vi "Put_Tracks_To_FRM-FRM_Matrix-3.vi"(2 "error IN":errorcluster, 3 "[IN] Matrix for Estimation \nSizes of Frame-to-Frame \nDisplacements from Tracks":dbl[][](array[numeric]), 5 "[IN] Tracks w/t Problems":T1(array[cluster])) -> (0 "error OUT":errorcluster, 1 "[OUT] Frame-to-Frame\nDisplacements Extract\nFrom Tracks":dbl[][](array[numeric]))   [LabVIEW 2013]
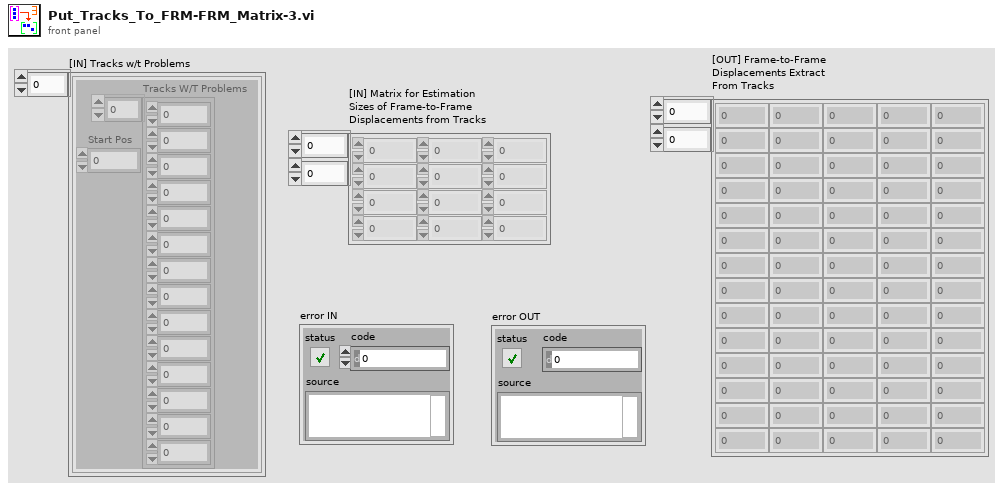
[diagram p1: front panel]
types:
  T1 = cluster{"Tracks W/T Problems":dbl[], "Start Pos":i32}[]
  T2 = cluster{"Tracks W/T Problems":dbl[], "Start Pos":i32}
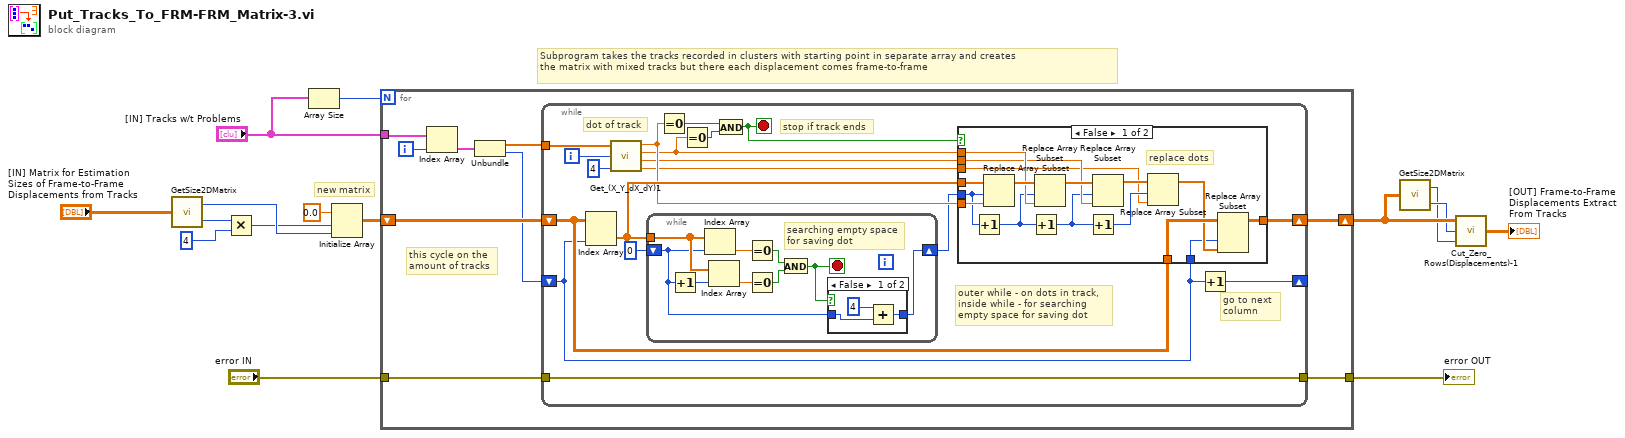
[diagram p0: block diagram]
diagram:
  # "Subprogram takes the tracks recorded in clusters with starting point in separate array and creates \nthe matrix with mixed tracks but there each displacement comes frame-to-frame"
  # "new matrix"
  n1 = call "GetSize2DMatrix.vi"("Array IN (2D)"="[IN] Matrix for Estimation \nSizes of Frame-to-Frame \nDisplacements from Tracks") -> ("# Cols"=w4:i32, "# Rows"=w3:i32)
  n2 = Multiply(x=w3, y=4 ("x")) -> (x*y=w1:i32)
  n3 = Array Size(array="[IN] Tracks w/t Problems") -> (size(s)=w8:i32)
  n4 = Initialize Array(0.0 ("element"), w1, w4) -> (w14:dbl[][])
  n5 = for {
    N: w8 -> [_]
    shift-right: [w23] -> w13
    shift-left: w14 -> [w24]
    tunnel: "[IN] Tracks w/t Problems" -> [w22]
    tunnel: "error IN" -> [w17]
    tunnel: [w16] -> w5
    i -> [w21]
    # "this cycle on the \namount of tracks"
    n6 = Index Array(array=w22, index=w21) -> (element=w20:T2)
    n7 = Unbundle(w20) -> ("Tracks W/T Problems"=w19:dbl[], "Start Pos"=w18:i32)
    n8 = while {
      tunnel: w19 -> [w42]
      shift-right: [w29] -> w23
      shift-left: w24 -> [w30]
      shift-right: [w27] -> _
      shift-left: w18 -> [w28]
      tunnel: w17 -> [w25]
      tunnel: [w25] -> w16
      i -> [w41]
      stop <- w26 stop-if-true
      # "outer while - on dots in track,\ninside while - for searching \nempty space for saving dot"
      # "go to next \ncolumn"
      # "stop if track ends"
      # "dot of track"
      n9 = Index Array(array=w30, index (col)=w28) -> (element=w36:dbl[])  [unwired: 1 in]
      n10 = call "Get_(X_Y_dX_dY)1.vi"("(X,Y,dX,dY)"=w42, "index"=w41, "multiplier"=4 ("multiplayer")) -> ("X"=w35:dbl, "Y"=w33:dbl, "dX"=w32:dbl, "dY"=w31:dbl)
      n11 = while {
        tunnel: w36 -> [w66]
        shift-right: [w60] -> w34
        shift-left: 0 -> [w61]
        stop <- w62 stop-if-true
        # "searching empty space\nfor saving dot"
        n12 = Increment(x=w61) -> (x+1=w67:i32)
        n13 = Index Array(array=w66, index=w61) -> (element=w68:dbl)
        n14 = Index Array(array=w66, index=w67) -> (element=w65:dbl)
        n15 = Equal To 0?(x=w68) -> (x = 0?=w64:bool)
        n16 = Equal To 0?(x=w65) -> (x = 0?=w63:bool)
        n17 = And(x=w64, y=w63) -> (x .and. y?=w62:bool)
        n18 = case shown="False" w62 {
          tunnel: w61 -> [w70 w72]
          tunnel: [w71 w72] -> w60
          frame False {
            n19 = Add(x=4, y=w70) -> (x+y=w71:i32)
          }
          frame True {
          }
        }
      }
      n20 = Equal To 0?(x=w35) -> (x = 0?=w39:bool)
      n21 = Equal To 0?(x=w33) -> (x = 0?=w38:bool)
      n22 = And(x=w39, y=w38) -> (x .and. y?=w26:bool)
      n23 = case shown="False" w26 {
        tunnel: w36 -> [w58 _]
        tunnel: w35 -> [w57 _]
        tunnel: w34 -> [w55 _]
        tunnel: w33 -> [w54 _]
        tunnel: w32 -> [w51 _]
        tunnel: w31 -> [w47 _]
        tunnel: w30 -> [w46 w59]
        tunnel: [w44 w59] -> w29
        tunnel: w28 -> [w43 _]
        frame False {
          # "replace dots"
          n24 = Increment(x=w55) -> (x+1=w52:i32)
          n25 = Replace Array Subset(array=w58, new element=w57, index=w55) -> (w56:dbl[])
          n26 = Increment(x=w52) -> (x+1=w49:i32)
          n27 = Replace Array Subset(array=w56, new element=w54, index=w52) -> (w53:dbl[])
          n28 = Increment(x=w49) -> (x+1=w48:i32)
          n29 = Replace Array Subset(array=w53, new element=w51, index=w49) -> (w50:dbl[])
          n30 = Replace Array Subset(array=w50, new element=w47, index=w48) -> (w45:dbl[])
          n31 = Replace Array Subset(array=w46, new element=w45, index (col)=w43) -> (w44:dbl[][])  [unwired: 1 in]
        }
        frame True {
        }
      }
      n32 = Increment(x=w28) -> (x+1=w27:i32)
    }
  }
  "error OUT" <- w5
  n33 = call "GetSize2DMatrix.vi"("Array IN (2D)"=w13) -> ("# Cols"=w11:i32, "# Rows"=w12:i32)
  n34 = call "Cut_Zero_Rows(Displacements)-1.vi"("# Cols"=w11, "# Rows"=w12, "Array IN"=w13) -> ("Array OUT"=→"[OUT] Frame-to-Frame\nDisplacements Extract\nFrom Tracks":dbl[][])
